vi "TestLocalizeLooped.vi"() -> ()   [LabVIEW 2011]
uses:
  JelmersTracker.llb/TrackerDLL.vi
panel:
  in  "profileWidth":i32=32
  out "ZLUT":sgl[][](graph)
  out "Intensity Graph":sgl[][](graph)
  in  "image size":cluster{"width":u32, "height":u32}={"width"=150, "height"=150}
  in  "Z random factor":dbl
  in  "z center":dbl=0.5
  out "Z localization":dbl(graph)
  in  "x scalefactor":sgl=0.1
  out "X Chart":dbl(graph)
  in  "jump period":i32=20
  in  "XCorWindow":u32=128
  in  "maxphotoncount":sgl=50000.0
  in  "Max Z":sgl=6.0
  in  "Min Z":sgl=1.0
  in  "Z planes":i32=60
  out "FPS":dbl
  out "Loop count":i32
  out "appended path":path
  in  "Show graphs":bool
  in  "Use debug library":bool
  in  "xcor_iterations":i32=2
  out "X profile":sgl[](graph)
  out "Y profile":sgl[](graph)
  out "Y result":sgl[](graph)
  out "True Y":dbl
  out "True X":dbl
  out "COM results":cluster{dbl, dbl}(graph)
  out "XCor results":cluster{dbl, dbl}(graph)
  in  "y center":dbl=75.0
  in  "x center":dbl=75.0 min=40.0 max=200.0
  out "X result":sgl[](graph)
  in  "Stop loop":bool
  out "median":sgl
  out "xcorpos":cluster{"XCor X":sgl, "XCor Y":sgl}
  out "COM":cluster{"comX":sgl, "comY":sgl}
  out "Image":T1(plugin-control)
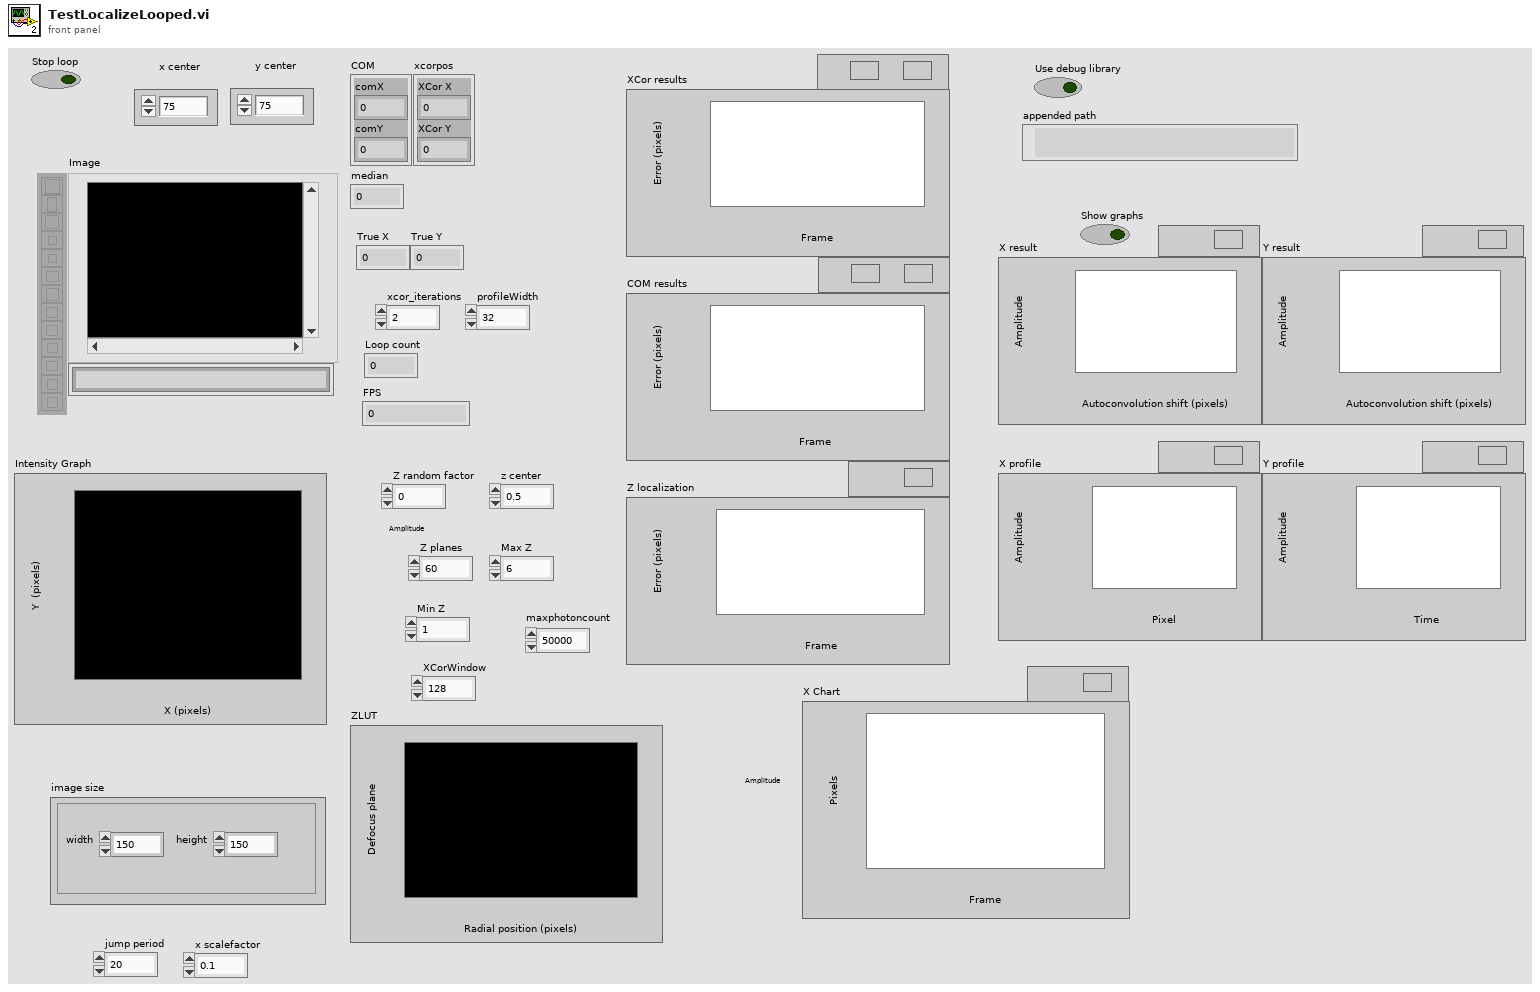
[diagram p1: front panel]
types:
  T1 = typedef "IMAQ Image.ctl" = refnum<image>
  T2 = typedef "Image Type" = u32
  T3 = typedef "TrackerInstance.ctl" = cluster{"Tracker Pointer":u64, "Image size":cluster{"width":u32, "height":u32}}
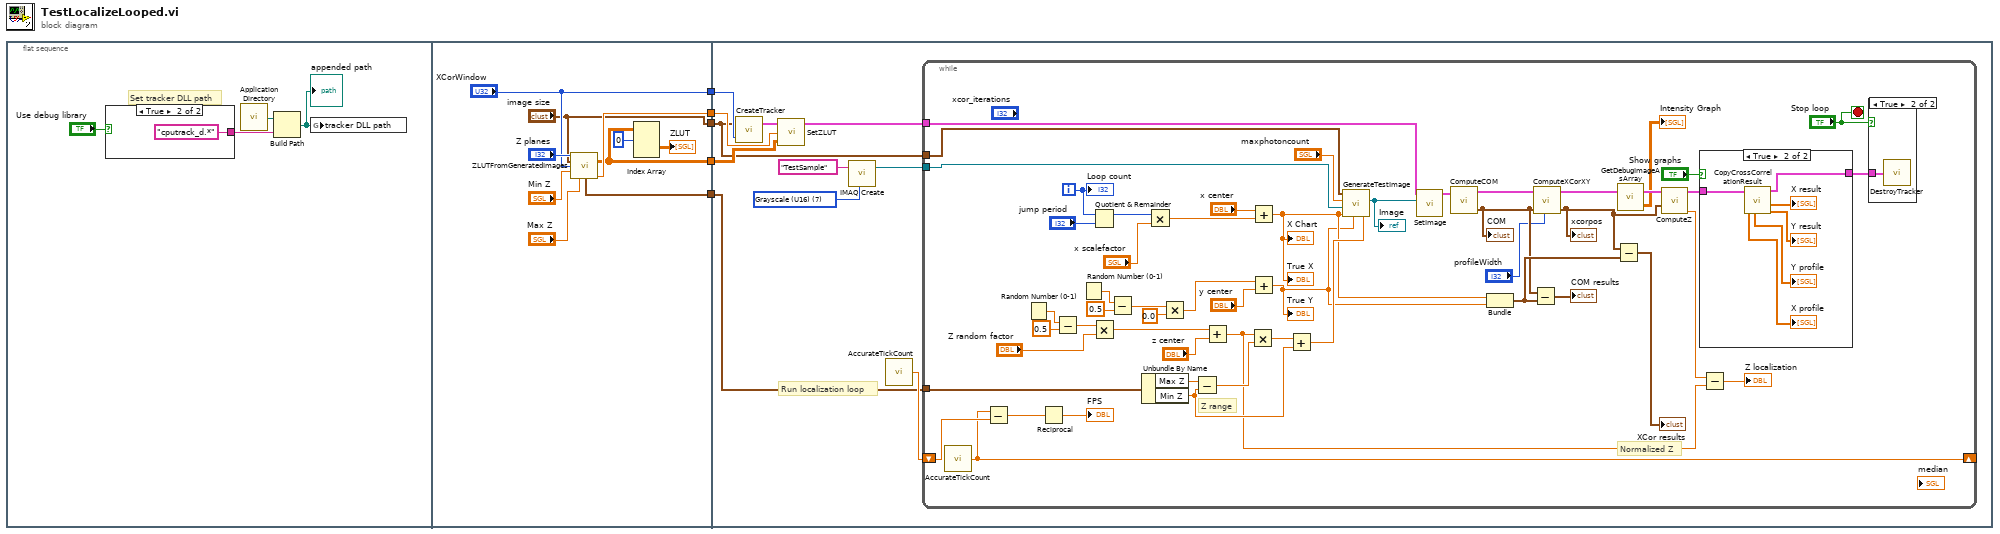
[diagram p0: block diagram]
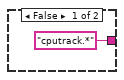
[diagram p2: hidden frame]
diagram:
  n1 = flat-sequence {
    tunnel: [w20] -> w5
    tunnel: ["image size"] -> w4
    tunnel: ["XCorWindow"] -> w3
    tunnel: [w16] -> w2
    tunnel: [w12] -> w1
    tunnel: w5 -> [w31]
    tunnel: w4 -> [w24]
    tunnel: w3 -> [w30]
    tunnel: w2 -> [w26]
    tunnel: w1 -> [w25]
    frame #0 {
      # "Set tracker DLL path"
      n2 = case shown="True" "Use debug library" {
        tunnel: ["cputrack.*" "cputrack_d.*"] -> w7
        frame False {
        }
        frame True {
        }
      }
      n3 = call <vilib>:"Application Directory.vi"() -> ("Application Directory"=w6:path)
      n4 = Build Path(base path=w6, name or relative path=w7) -> (appended path=w8:path)
      "appended path" <- w8
      n5 = global write "TrackerDLL.vi" "tracker DLL path"(w8) -> ()
    }
    frame #1 {
      n6 = call "ZLUTFromGeneratedImages.vi"("Z planes"="Z planes", "Image size"="image size", "XCorWindow"="XCorWindow", "Min Z"="Min Z", "Max Z"="Max Z") -> ("ZLUT"=w12:sgl[][][], "z range"=w20:cluster{"Min Z":sgl, "Max Z":sgl}, "radius"=w16:sgl)  [unwired: 8 in]
      n7 = Index Array(array=w12, index (dim 0)=0 ("index (page)")) -> (element=→"ZLUT":sgl[][])  [unwired: 2 in]
    }
    frame #2 {
      w29 = T2 7 items=["Grayscale (U8)", "Grayscale (I16)", "Grayscale (SGL)", "Complex (CSG)", "RGB (U32)", "HSL (U32)", "RGB (U64)", "Grayscale (U16)"] ("Image Type")
      # "Run localization loop"
      n8 = call "CreateTracker.vi"("XCorWindow"=w30, "Image size"=w24) -> ("tracker"=w23:T3)  [unwired: 1 in]
      n9 = call "SetZLUT.vi"("zlut"=w25, "profile_radius"=w26, "tracker instance"=w23) -> ("tracker"=w22:T3)  [unwired: 2 in]
      n10 = call "IMAQ Create"("Image Name"="TestSample" ("String"), "Image Type"=w29) -> ("New Image"=w27:T1)  [unwired: 3 in, 1 out]
      n11 = call "AccurateTickCount.vi"() -> ("seconds"=w32:dbl)
      n12 = while {
        tunnel: w22 -> [w35]
        tunnel: w27 -> [w85]
        shift-right: [w75] -> _
        shift-left: w32 -> [w76]
        tunnel: w24 -> [w72]
        tunnel: w31 -> [w60]
        i -> [w69]
        stop <- "Stop loop" stop-if-true
        # "Normalized Z"
        # "Z range"
        n13 = call "AccurateTickCount.vi"() -> ("seconds"=w75:dbl)
        n14 = Subtract(x=w75, y=w76) -> (x-y=w74:dbl)
        n15 = Random Number (0-1)() -> (number: 0 to 1=w62:dbl)
        n16 = Reciprocal(x=w74) -> (1/x=→"FPS":dbl)
        n17 = Subtract(x=w62, y=0.5) -> (x-y=w50:dbl)
        n18 = Random Number (0-1)() -> (number: 0 to 1=w81:dbl)
        n19 = Quotient & Remainder(x=w69, y="jump period") -> (x-y*floor(x/y)=w67:i32)  [unwired: 1 out]
        n20 = Multiply(x=w50, y="Z random factor") -> (x*y=w48:dbl)
        n21 = Subtract(x=w81, y=0.5) -> (x-y=w79:dbl)
        n22 = Unbundle By Name(w60) -> ("Max Z"=w59:sgl, "Min Z"=w56:sgl)
        n23 = Multiply(x=w67, y="x scalefactor") -> (x*y=w65:sgl)
        n24 = Multiply(x=w79, y=sgl 0.0) -> (x*y=w83:dbl)
        n25 = Subtract(x=w59, y=w56) -> (x-y=w57:sgl)
        n26 = Add(x=w48, y="z center") -> (x+y=w52:dbl)
        n27 = Multiply(x=w52, y=w57) -> (x*y=w55:dbl)
        n28 = Add(x="x center", y=w65) -> (x+y=w47:dbl)
        "True X" <- w47
        "X Chart" <- w47
        n29 = Add(x=w83, y="y center") -> (x+y=w46:dbl)
        "True Y" <- w46
        n30 = Add(x=w55, y=w56) -> (x+y=w54:dbl)
        n31 = call "GenerateTestImage.vi"("spotsize"=w54, "ypos"=w46, "xpos"=w47, "image"=w85, "maxphotoncount"="maxphotoncount", "Image size"=w72) -> ("Image"=w36:T1)  [unwired: 3 in]
        "Image" <- w36
        n32 = call "SetImage.vi"("Image"=w36, "tracker"=w35) -> ("tracker"=w34:T3)  [unwired: 5 in]
        n33 = call "ComputeCOM.vi"("tracker"=w34) -> ("tracker"=w40:T3, "position"=w37:cluster{"X":sgl, "Y":sgl})  [unwired: 2 in]
        "COM" <- w37
        n34 = Bundle(w47, w46) -> (w45:cluster{dbl, dbl})  [unwired: 1 in]
        n35 = Subtract(x=w37, y=w45) -> (x-y=→"COM results":cluster{dbl, dbl})
        n36 = call "ComputeXCorXY.vi"("tracker"=w40, "position"=w37, "profileWidth"="profileWidth") -> ("tracker"=w39:T3, "position"=w38:cluster{"X":sgl, "Y":sgl})  [unwired: 2 in, 1 out]
        "xcorpos" <- w38
        n37 = Subtract(x=w38, y=w45) -> (x-y=→"XCor results":cluster{dbl, dbl})
        n38 = call "GetDebugImageAsArray.vi"("tracker"=w39) -> ("image"=→"Intensity Graph":sgl[][], "tracker"=w42:T3)  [unwired: 1 in]
        n39 = call "ComputeZ.vi"("position"=w38, "tracker instance"=w42) -> ("Z"=w53:sgl, "tracker instance"=w64:T3)  [unwired: 4 in]
        n40 = case shown="True" "Show graphs" {
          tunnel: w64 -> [w86 w87]
          tunnel: [w86 w92] -> w78
          frame False {
          }
          frame True {
            n41 = call "CopyCrossCorrelationResult.vi"("tracker"=w87) -> ("x prof"=→"X profile":sgl[], "y prof"=→"Y profile":sgl[], "tracker"=w92:T3, "x result"=→"X result":sgl[], "y_result"=→"Y result":sgl[])  [unwired: 3 in]
          }
        }
        n42 = Subtract(x=w53, y=w52) -> (x-y=→"Z localization":dbl)
        n43 = case shown="True" "Stop loop" {
          tunnel: w78 -> [_ w93]
          frame False {
          }
          frame True {
            n44 = call "DestroyTracker.vi"("tracker instance"=w93) -> ()
          }
        }
        "Loop count" <- w69
      }
    }
  }
